vi "AMZ_S3_APIHLP_Parse ACP to XML.vi"(8 "error in (no error)":errorcluster, 11 "AccessControlPolicy":T1) -> (0 "error out":errorcluster, 3 "ACP XML String":string)   [LabVIEW 2015, in "LV Interface for Amazon S3.lvlib"]
uses:
  LV Interface for Amazon S3.lvlib
  Typedefs/AMZ_S3_API_AccessControlPolicy.ctl
  Typedefs/AMZ_S3_API_Owner.ctl
  Typedefs/AMZ_S3_API_Bucket ACL Permission.ctl
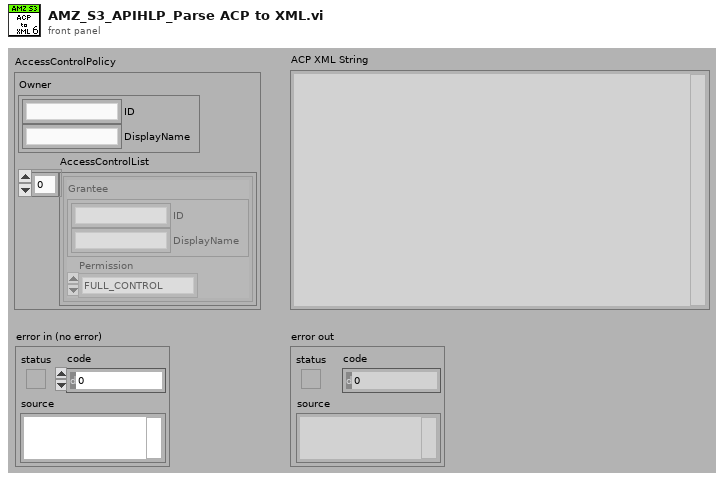
[diagram p1: front panel]
types:
  T1 = typedef "LV Interface for Amazon S3.lvlib/AMZ_S3_API_AccessControlPolicy.ctl" = cluster{"Owner":T2, "AccessControlList":cluster{"Grantee":T2, "Permission":T3}[]}
  T2 = typedef "LV Interface for Amazon S3.lvlib/AMZ_S3_API_Owner.ctl" = cluster{"ID":string, "DisplayName":string}
  T3 = typedef "LV Interface for Amazon S3.lvlib/AMZ_S3_API_Bucket ACL Permission.ctl" = enum16{"FULL_CONTROL", "WRITE", "WRITE_ACP", "READ", "READ_ACP"}
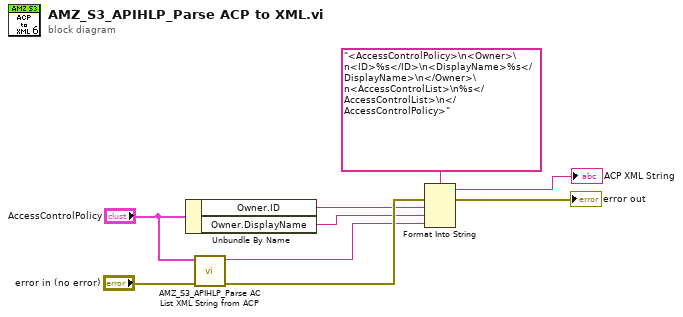
[diagram p0: block diagram]
diagram:
  n1 = Unbundle By Name("AccessControlPolicy") -> ("Owner.ID"=w5:string, "Owner.DisplayName"=w4:string)
  n2 = call "AMZ_S3_APIHLP_Parse AC List XML String from ACP.vi"("error in (no error)"="error in (no error)", "AccessControlPolicy"="AccessControlPolicy") -> ("error out"=w6:errorcluster, "AccessControlList XML"=w3:string)  [unwired: 8 in]
  n3 = Format Into String(format string="<AccessControlPolicy>\n<Owner>\n<ID>%s</ID>\n<DisplayName>%s</DisplayName>\n</Owner>\n<AccessControlList>\n%s</AccessControlList>\n</AccessControlPolicy>", error in=w6, w5, w4, w3) -> (resulting string=→"ACP XML String":string, error out=→"error out":errorcluster)  [unwired: 1 in]
